vi "DSF.Engine.Timing.Create.vi"(8 "error in (no error)":errorcluster, 9 "Offset":u64, 10 "Decimation":u64=1, 11 "Priority":u64) -> (0 "error out":errorcluster, 3 "Timing":refnum<class "DSF.Engine.Timing.lvclass">)   [LabVIEW 2017, in "DSF.Engine.lvlib" / "DSF.Engine.Timing.lvclass"]
uses:
  DSF.Engine.Timing.lvclass
  DSF.Engine.Timing.lvclass/DSF.Engine.Timing.ctl
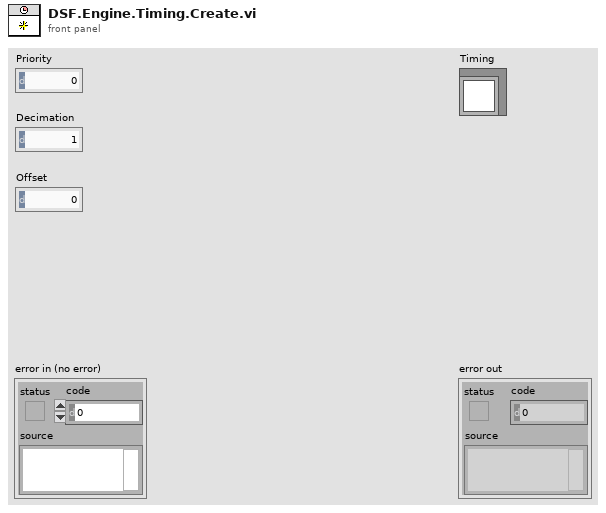
[diagram p1: front panel]
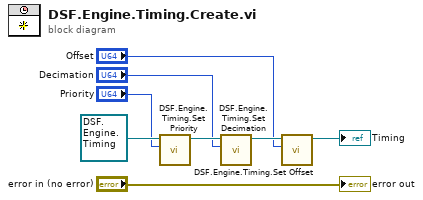
[diagram p0: block diagram]
diagram:
  n1 = call "DSF.Engine.Timing.Set Priority.vi"("Priority"="Priority", "Timing in"=refnum<class "DSF.Engine.Timing.lvclass"> refnum ("Timing")) -> ("Timing out"=w6:refnum<class "DSF.Engine.Timing.lvclass">)  [unwired: 9 in]
  n2 = call "DSF.Engine.Timing.Set Decimation.vi"("Decimation"="Decimation", "Timing in"=w6) -> ("Timing out"=w4:refnum<class "DSF.Engine.Timing.lvclass">)  [unwired: 9 in]
  n3 = call "DSF.Engine.Timing.Set Offset.vi"("Offset"="Offset", "Timing in"=w4) -> ("Timing out"=→"Timing":refnum<class "DSF.Engine.Timing.lvclass">)  [unwired: 9 in]
  "error out" <- "error in (no error)"
